vi "Begin.vi"(8 "error in":errorcluster) -> (0 "error out":errorcluster)   [LabVIEW 2017]
doc: "Called before other user functions, this VI is expected to open initial I/O refnums, load in file data, and do all program initialization. Notice that the <B>error out</B> terminal is simply used for data flow. Wiring it to other structures or subVIs ensures that this VI runs first."
uses:
  <vilib>/Rock Robotics/WPI/DriverStation/WPI_DriverStationRobotMode2.ctl
  <vilib>/Rock Robotics/WPI/Joystick/WPI_JoystickDeviceEnum.ctl
  <vilib>/Rock Robotics/SystemInterfaces/DIO/FPGA_DIOChannel.ctl
  Phoenix-LabVIEW/Motor Controller/Controls/CTRE_Phoenix_MotorControl_FeedbackDevice.ctl
  Robot Global Data.vi
  <vilib>/Rock Robotics/Network Tables/NT Write String Array.vi
  <vilib>/Rock Robotics/Network Tables/NT Write Number.vi
  <vilib>/Rock Robotics/WPI/Counter/WPI_CounterDigitalInputToDigitalSource.vi
panel:
  in  "DriveRamp":dbl=0.7 format="%#_13g"
  in  "LiftRamp":dbl=0.5 format="%#_13g"
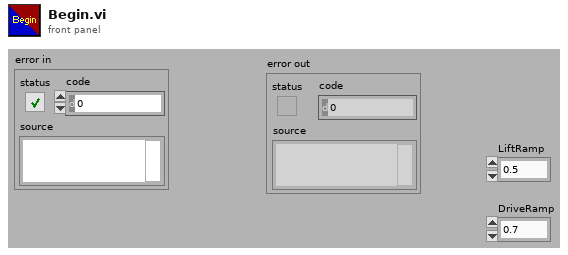
[diagram p1: front panel]
types:
  T1 = typedef "CTRE_Phoenix_MotorControl_FeedbackDevice.ctl" = i8
  T2 = typedef "FPGA_DIOChannel.ctl" = enum8{"DIO 0", "DIO 1", "DIO 2", "DIO 3", "DIO 4", "DIO 5", "DIO 6", "DIO 7", "DIO 8", "DIO 9", "DIO MXP 0", "DIO MXP 1", "DIO MXP 2", "DIO MXP 3", "DIO MXP 4", "DIO MXP 5", "DIO MXP 6", "DIO MXP 7", "DIO MXP 8", "DIO MXP 9", "DIO MXP 10", "DIO MXP 11", "DIO MXP 12", "DIO MXP 13", "DIO MXP 14", "DIO MXP 15", "SPI Port CS1", "SPI Port CS2", "SPI Port CS3", "SPI Port MISO", "SPI Port MOSI", "Invalid"}
  T3 = typedef "WPI_JoystickDeviceEnum.ctl" = enum16{"USB 0", "USB 1", "USB 2", "USB 3", "USB 4", "USB 5"}
  T4 = typedef "WPI_DriverStationRobotMode2.ctl" = enum16{"Autonomous Disabled", "Autonomous Enabled", "Teleop Disabled", "Teleop Enabled", "Disconnected", "Finish", "Test Disabled", "Test Enabled", "Emergency Stopped"}
  T5 = typedef "WPI_MotorControlDeviceRef.ctl" = cluster{"DeviceStatus":errorcluster, "Type":T6, "PWM":cluster{"PWM Channel":T7, "DeadBand":T8}, "CAN":cluster{"Device Number":u8, "SetOutput VI Ref":variant, "GetOutput VI Ref":variant, "Enable VI Ref":variant, "Disable VI Ref":variant, "Data":variant}, "Invert":bool, "DIO PWM":cluster{"PWM \"Enable\" Channel":T7, "DIOChannel":T2, "PWM Rate":dbl}}
  T6 = typedef "WPI_MotorControlType.ctl" = enum16{"PWM", "CAN", "DIO PWM"}
  T7 = typedef "FPGA_DIOPWMChannel.ctl" = enum8{"PWM 0", "PWM 1", "PWM 2", "PWM 3", "PWM 4", "PWM 5", "PWM 6", "PWM 7", "PWM 8", "PWM 9", "PWM MXP 0", "PWM MXP 1", "PWM MXP 2", "PWM MXP 3", "PWM MXP 4", "PWM MXP 5", "PWM MXP 6", "PWM MXP 7", "PWM MXP 8", "PWM MXP 9", "Invalid"}
  T8 = typedef "WPI_PWMDeadband.ctl" = cluster{"Name":string, "maxPositivePwm":i32, "minPositivePwm":i32, "centerPwm":i32, "maxNegativePwm":i32, "minNegativePwm":i32, "angularRange":u16}
  T9 = typedef "WPI_JoystickDevRef.ctl" = cluster{"Device":T3}
  T10 = typedef "WPI_DigitalInputDevRef.ctl" = cluster{"DevStatus":errorcluster, "DIO Channel":T2}
  T11 = typedef "FPGA_CounterEncoderSourceConvertionLVSourceType.ctl" = cluster{"DevStatus":errorcluster, "AnalogTriggerMode?":bool, "DigitalMode":cluster{"DIO Channel":T12}, "AnalogTriggerMode":cluster{"AnalogTriggerIndex":T13, "OutputType":T14}}
  T12 = typedef "FPGA_DIODigitalSourceChannel.ctl" = enum8{"DIO 0", "DIO 1", "DIO 2", "DIO 3", "DIO 4", "DIO 5", "DIO 6", "DIO 7", "DIO 8", "DIO 9", "DIO MXP 0", "DIO MXP 1", "DIO MXP 2", "DIO MXP 3", "DIO MXP 4", "DIO MXP 5", "DIO MXP 6", "DIO MXP 7", "DIO MXP 8", "DIO MXP 9", "DIO MXP 10", "DIO MXP 11", "DIO MXP 12", "DIO MXP 13", "DIO MXP 14", "DIO MXP 15", "Disabled"}
  T13 = typedef "FPGA_AnalogTriggerIndex.ctl" = enum8{"Trig 0", "Trig 1", "Trig 2", "Trig 3", "Trig 4", "Trig 5", "Trig 6", "Trig 7", "Invalid"}
  T14 = typedef "FPGA_AnalogTriggerOutType.ctl" = enum16{"InWindow", "TriggerState", "Rising", "Falling"}
  T15 = typedef "WPI_EncoderDevRef.ctl" = cluster{"DevStatus":errorcluster, "EncoderIndex":T16, "CounterIndex":T17, "DistancePerCount":dbl, "Decoding Type":T18}
  T16 = typedef "FPGA_EncoderIdx.ctl" = enum8{"Enc 0", "Enc 1", "Enc 2", "Enc 3", "Enc 4", "Enc 5", "Enc 6", "Enc 7", "Invalid"}
  T17 = typedef "FPGA_CounterCtrSystemIndex.ctl" = enum8{"Ctr 0", "Ctr 1", "Ctr 2", "Ctr 3", "Ctr 4", "Ctr 5", "Ctr 6", "Ctr 7", "Invalid"}
  T18 = typedef "WPI_EncoderType.ctl" = enum16{"1x", "2x", "4x"}
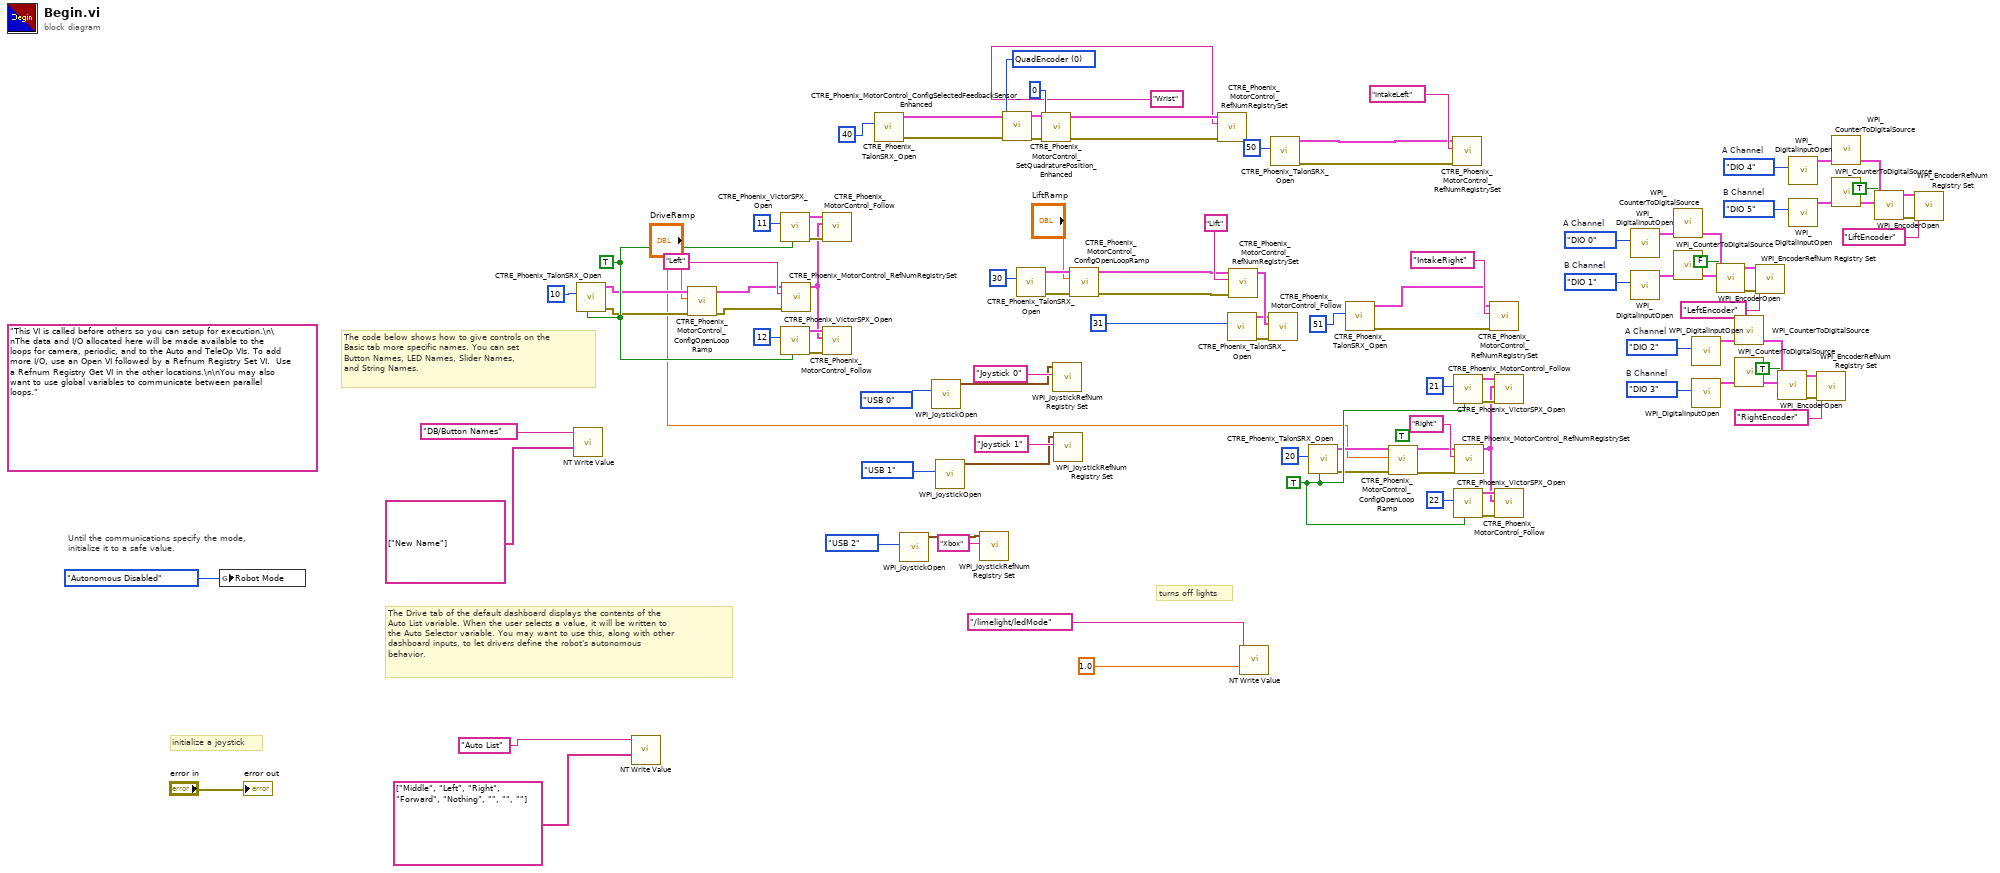
[diagram p0: block diagram]
diagram:
  w20 = T1 0 items=["None"=-1, "QuadEncoder"=0, "Analog"=2, "Tachometer"=4, "Pulse Width Encoded Position"=8, "Sensor Sum (S0 + S1)"=9, "Sensor Difference (D0 - D1)"=10, "Remote Source 0"=11, "Remote Source 1"=12, "Software Emulated"=15] ("Feedback Device")
  w34 = FPGA_DIOChannel."DIO 5"  # B Channel
  w33 = FPGA_DIOChannel."DIO 4"  # A Channel
  (unwired) TRUE ("Enable Current Limit?")
  w40 = TRUE
  w47 = TRUE ("Invert")
  w56 = FPGA_DIOChannel."DIO 3"  # B Channel
  w55 = FPGA_DIOChannel."DIO 2"  # A Channel
  w65 = FPGA_DIOChannel."DIO 1"  # B Channel
  w64 = FPGA_DIOChannel."DIO 0"  # A Channel
  (unwired) "This VI is called before others so you can setup for execution.\n\nThe data and I/O allocated here will be made available to the loops for camera, periodic, and to the Auto and TeleOp VIs. To add more I/O, use an Open VI followed by a Refnum Registry Set VI.  Use a Refnum Registry Get VI in the other locations.\n\nYou may also want to use global variables to communicate between parallel loops."
  # "turns off lights"
  # "The Drive tab of the default dashboard displays the contents of the\nAuto List variable. When the user selects a value, it will be written to\nthe Auto Selector variable. You may want to use this, along with other\ndashboard inputs, to let drivers define the robot's autonomous\nbehavior."
  # "The code below shows how to give controls on the\nBasic tab more specific names. You can set\nButton Names, LED Names, Slider Names,\nand String Names."
  # "initialize a joystick"
  # "Until the communications specify the mode,\ninitialize it to a safe value."
  n1 = global write "Robot Global Data.vi" "Robot Mode"(WPI_DriverStationRobotMode2."Autonomous Disabled" ("Robot Mode")) -> ()
  n2 = call-poly <vilib>:"NT Write Value.vi"("String Array"=string[] ["New Name"], "Name"="DB/Button Names") -> ()  [unwired: 9 in, 1 out]
  n3 = call <vilib>:"CTRE_Phoenix_TalonSRX_Open.vi"("Invert"=w40, "Device Number"=u8 10) -> ("error out"=w16:errorcluster, "CAN Talon SRX Ref"=w17:T5)  [unwired: 8 in]
  n4 = call-poly <vilib>:"NT Write Value.vi"("String Array"=string[] ["Middle", "Left", "Right", "Forward", "Nothing", "", "", ""], "Name"="Auto List") -> ()  [unwired: 9 in, 1 out]
  n5 = call "CTRE_Phoenix_MotorControl_ConfigOpenLoopRamp.vi"("error in (no error)"=w16, "secondsFromNeutralToFull"="DriveRamp", "PhoenixMotorControlDevRef"=w17) -> ("error out"=w15:errorcluster, "PhoenixMotorControlDevRef"=w18:T5)  [unwired: 7 in]
  n6 = call "CTRE_Phoenix_VictorSPX_Open.vi"("Invert"=w40, "Device Number"=u8 11) -> ("error out"=w95:errorcluster, "CAN Talon SRX Ref"=w94:T5)  [unwired: 8 in]
  n7 = call "CTRE_Phoenix_VictorSPX_Open.vi"("Invert"=w40, "Device Number"=u8 12) -> ("error out"=w93:errorcluster, "CAN Talon SRX Ref"=w92:T5)  [unwired: 8 in]
  n8 = call "CTRE_Phoenix_MotorControl_RefNumRegistrySet.vi"("error in (no error)"=w15, "refnum name"="Left", "PhoenixMotorControlDevRef"=w18) -> ("PhoenixMotorControlDevRef"=w79:T5)  [unwired: 7 in, 1 out]
  n9 = call "CTRE_Phoenix_MotorControl_Follow.vi"("error in (no error)"=w95, "Master Controller to Follow"=w79, "PhoenixMotorControlDevRef"=w94) -> ()  [unwired: 7 in, 2 out]
  n10 = call "CTRE_Phoenix_MotorControl_Follow.vi"("error in (no error)"=w93, "Master Controller to Follow"=w79, "PhoenixMotorControlDevRef"=w92) -> ()  [unwired: 7 in, 2 out]
  n11 = call <vilib>:"CTRE_Phoenix_TalonSRX_Open.vi"("Device Number"=u8 40) -> ("error out"=w5:errorcluster, "CAN Talon SRX Ref"=w6:T5)  [unwired: 9 in]
  n12 = call <vilib>:"WPI_JoystickOpen.vi"("JoystickDevice"=WPI_JoystickDeviceEnum."USB 2") -> ("JoystickDevRef"=w44:T9)  [unwired: 10 in]
  n13 = call <vilib>:"WPI_JoystickOpen.vi"("JoystickDevice"=WPI_JoystickDeviceEnum."USB 0") -> ("JoystickDevRef"=w35:T9)  [unwired: 10 in]
  n14 = call <vilib>:"WPI_JoystickOpen.vi"("JoystickDevice"=WPI_JoystickDeviceEnum."USB 1") -> ("JoystickDevRef"=w36:T9)  [unwired: 10 in]
  n15 = call <vilib>:"WPI_JoystickRefNum Registry Set.vi"("refnum name"="Xbox", "JoystickDevRef"=w44) -> ()  [unwired: 8 in, 2 out]
  n16 = call "CTRE_Phoenix_MotorControl_ConfigSelectedFeedbackSensor_Enhanced.vi"("error in (no error)"=w5, "Feedback Device"=w20, "PhoenixMotorControlDevRef"=w6) -> ("error out"=w21:errorcluster, "PhoenixMotorControlDevRef"=w22:T5)  [unwired: 7 in]
  n17 = call <vilib>:"CTRE_Phoenix_TalonSRX_Open.vi"("Device Number"=u8 30) -> ("error out"=w42:errorcluster, "CAN Talon SRX Ref"=w43:T5)  [unwired: 9 in]
  n18 = call <vilib>:"CTRE_Phoenix_MotorControl_SetQuadraturePosition_Enhanced.vi"("error in (no error)"=w21, "New Position"=0, "PhoenixMotorControlDevRef"=w22) -> ("error out"=w8:errorcluster, "PhoenixMotorControlDevRef"=w9:T5)  [unwired: 7 in]
  n19 = call <vilib>:"WPI_JoystickRefNum Registry Set.vi"("refnum name"="Joystick 0", "JoystickDevRef"=w35) -> ()  [unwired: 8 in, 2 out]
  n20 = call <vilib>:"WPI_JoystickRefNum Registry Set.vi"("refnum name"="Joystick 1", "JoystickDevRef"=w36) -> ()  [unwired: 8 in, 2 out]
  n21 = call "CTRE_Phoenix_MotorControl_ConfigOpenLoopRamp.vi"("error in (no error)"=w42, "secondsFromNeutralToFull"="LiftRamp", "PhoenixMotorControlDevRef"=w43) -> ("error out"=w23:errorcluster, "PhoenixMotorControlDevRef"=w24:T5)  [unwired: 7 in]
  n22 = call "CTRE_Phoenix_MotorControl_RefNumRegistrySet.vi"("error in (no error)"=w8, "refnum name"="Wrist", "PhoenixMotorControlDevRef"=w9) -> ()  [unwired: 7 in, 2 out]
  n23 = call <vilib>:"CTRE_Phoenix_TalonSRX_Open.vi"("Device Number"=u8 31) -> ("error out"=w73:errorcluster, "CAN Talon SRX Ref"=w74:T5)  [unwired: 9 in]
  n24 = call "CTRE_Phoenix_MotorControl_RefNumRegistrySet.vi"("error in (no error)"=w23, "refnum name"="Lift", "PhoenixMotorControlDevRef"=w24) -> ("PhoenixMotorControlDevRef"=w75:T5)  [unwired: 7 in, 1 out]
  n25 = call-poly <vilib>:"NT Write Value.vi"("Numeric"=1.0, "Name"="/limelight/ledMode") -> ()  [unwired: 9 in, 1 out]
  n26 = call "CTRE_Phoenix_MotorControl_Follow.vi"("error in (no error)"=w73, "Master Controller to Follow"=w75, "PhoenixMotorControlDevRef"=w74) -> ()  [unwired: 7 in, 2 out]
  n27 = call <vilib>:"CTRE_Phoenix_TalonSRX_Open.vi"("Device Number"=u8 50) -> ("error out"=w3:errorcluster, "CAN Talon SRX Ref"=w4:T5)  [unwired: 9 in]
  n28 = call <vilib>:"CTRE_Phoenix_TalonSRX_Open.vi"("Invert"=w47, "Device Number"=u8 20) -> ("error out"=w12:errorcluster, "CAN Talon SRX Ref"=w13:T5)  [unwired: 8 in]
  n29 = call <vilib>:"CTRE_Phoenix_TalonSRX_Open.vi"("Device Number"=u8 51) -> ("error out"=w1:errorcluster, "CAN Talon SRX Ref"=w2:T5)  [unwired: 9 in]
  n30 = call "CTRE_Phoenix_MotorControl_ConfigOpenLoopRamp.vi"("error in (no error)"=w12, "secondsFromNeutralToFull"="DriveRamp", "PhoenixMotorControlDevRef"=w13) -> ("error out"=w11:errorcluster, "PhoenixMotorControlDevRef"=w14:T5)  [unwired: 7 in]
  n31 = call "CTRE_Phoenix_MotorControl_RefNumRegistrySet.vi"("error in (no error)"=w3, "refnum name"="IntakeLeft", "PhoenixMotorControlDevRef"=w4) -> ()  [unwired: 7 in, 2 out]
  n32 = call "CTRE_Phoenix_VictorSPX_Open.vi"("Invert"=w47, "Device Number"=u8 21) -> ("error out"=w87:errorcluster, "CAN Talon SRX Ref"=w86:T5)  [unwired: 8 in]
  n33 = call "CTRE_Phoenix_VictorSPX_Open.vi"("Invert"=w47, "Device Number"=u8 22) -> ("error out"=w85:errorcluster, "CAN Talon SRX Ref"=w84:T5)  [unwired: 8 in]
  n34 = call "CTRE_Phoenix_MotorControl_RefNumRegistrySet.vi"("error in (no error)"=w11, "refnum name"="Right", "PhoenixMotorControlDevRef"=w14) -> ("PhoenixMotorControlDevRef"=w78:T5)  [unwired: 7 in, 1 out]
  n35 = call "CTRE_Phoenix_MotorControl_RefNumRegistrySet.vi"("error in (no error)"=w1, "refnum name"="IntakeRight", "PhoenixMotorControlDevRef"=w2) -> ()  [unwired: 7 in, 2 out]
  n36 = call "CTRE_Phoenix_MotorControl_Follow.vi"("error in (no error)"=w87, "Master Controller to Follow"=w78, "PhoenixMotorControlDevRef"=w86) -> ()  [unwired: 7 in, 2 out]
  n37 = call "CTRE_Phoenix_MotorControl_Follow.vi"("error in (no error)"=w85, "Master Controller to Follow"=w78, "PhoenixMotorControlDevRef"=w84) -> ()  [unwired: 7 in, 2 out]
  n38 = call <vilib>:"WPI_DigitalInputOpen.vi"("DIO Channel"=w64) -> ("DigitalInputDevRef"=w61:T10)  [unwired: 1 in, 9 out]
  n39 = call <vilib>:"WPI_DigitalInputOpen.vi"("DIO Channel"=w65) -> ("DigitalInputDevRef"=w62:T10)  [unwired: 1 in, 9 out]
  n40 = call-poly <vilib>:"WPI_CounterToDigitalSource.vi"("DigitalInputDevRef"=w61) -> ("Digital Source"=w60:T11)  [unwired: 6 out]
  n41 = call-poly <vilib>:"WPI_CounterToDigitalSource.vi"("DigitalInputDevRef"=w62) -> ("Digital Source"=w63:T11)  [unwired: 6 out]
  n42 = call <vilib>:"WPI_DigitalInputOpen.vi"("DIO Channel"=w55) -> ("DigitalInputDevRef"=w52:T10)  [unwired: 1 in, 9 out]
  n43 = call <vilib>:"WPI_DigitalInputOpen.vi"("DIO Channel"=w56) -> ("DigitalInputDevRef"=w53:T10)  [unwired: 1 in, 9 out]
  n44 = call <vilib>:"WPI_EncoderOpen.vi"("Invert Direction (False)"=FALSE, "BSource"=w63, "ASource"=w60) -> ("error out"=w59:errorcluster, "EncoderDevRef"=w58:T15)  [unwired: 5 in, 2 out]
  n45 = call-poly <vilib>:"WPI_CounterToDigitalSource.vi"("DigitalInputDevRef"=w52) -> ("Digital Source"=w51:T11)  [unwired: 6 out]
  n46 = call-poly <vilib>:"WPI_CounterToDigitalSource.vi"("DigitalInputDevRef"=w53) -> ("Digital Source"=w54:T11)  [unwired: 6 out]
  n47 = call <vilib>:"WPI_EncoderRefNum Registry Set.vi"("error in (no error)"=w59, "refnum name"="LeftEncoder", "EncoderDevRef"=w58) -> ()  [unwired: 7 in, 2 out]
  n48 = call <vilib>:"WPI_EncoderOpen.vi"("Invert Direction (False)"=TRUE, "BSource"=w54, "ASource"=w51) -> ("error out"=w50:errorcluster, "EncoderDevRef"=w49:T15)  [unwired: 5 in, 2 out]
  n49 = call <vilib>:"WPI_DigitalInputOpen.vi"("DIO Channel"=w33) -> ("DigitalInputDevRef"=w30:T10)  [unwired: 1 in, 9 out]
  n50 = call <vilib>:"WPI_DigitalInputOpen.vi"("DIO Channel"=w34) -> ("DigitalInputDevRef"=w31:T10)  [unwired: 1 in, 9 out]
  n51 = call <vilib>:"WPI_EncoderRefNum Registry Set.vi"("error in (no error)"=w50, "refnum name"="RightEncoder", "EncoderDevRef"=w49) -> ()  [unwired: 7 in, 2 out]
  n52 = call-poly <vilib>:"WPI_CounterToDigitalSource.vi"("DigitalInputDevRef"=w30) -> ("Digital Source"=w29:T11)  [unwired: 6 out]
  n53 = call-poly <vilib>:"WPI_CounterToDigitalSource.vi"("DigitalInputDevRef"=w31) -> ("Digital Source"=w32:T11)  [unwired: 6 out]
  n54 = call <vilib>:"WPI_EncoderOpen.vi"("Invert Direction (False)"=TRUE, "BSource"=w32, "ASource"=w29) -> ("error out"=w28:errorcluster, "EncoderDevRef"=w27:T15)  [unwired: 5 in, 2 out]
  n55 = call <vilib>:"WPI_EncoderRefNum Registry Set.vi"("error in (no error)"=w28, "refnum name"="LiftEncoder", "EncoderDevRef"=w27) -> ()  [unwired: 7 in, 2 out]
  "error out" <- "error in"
